vi "labview_master_02.vi"() -> ()   [LabVIEW 2018]
panel:
  out "Error Out 2":errorcluster caption="에러 출력"
  in  "Error In 2":errorcluster caption="에러 입력"
  out "Error Out":errorcluster caption="에러 출력"
  in  "Error In":errorcluster caption="에러 입력"
  in  "클러스터":cluster{"불리언":bool, "문자열":string, "숫자형 컨트롤":dbl}
  out "dimension 6":dbl[][][](array[numeric])
  out "dimension 5":dbl[][](array[numeric])
  out "dimension 4":dbl[](array[numeric])
  in  "dimension 3":dbl[][][](array[numeric])
  in  "dimension 2":dbl[][](array[numeric])
  in  "dimension 1":dbl[](array[numeric])
  in  "열거형":enum16{"Channel A", "Channel B", "Channel C"}(ring)
  in  "문자열":string
  in  "불리언":bool
  in  "정수":i32
  in  "부동소수점형":dbl
  # "사용자 인터페이스 구현"
  # "숫자"
  # "불리언"
  # "문자열"
  # "열거형"
  # "배열"
  # "클러스터"
  # "기본 클러스터"
  # "전부 control"
  # "module 만들기"
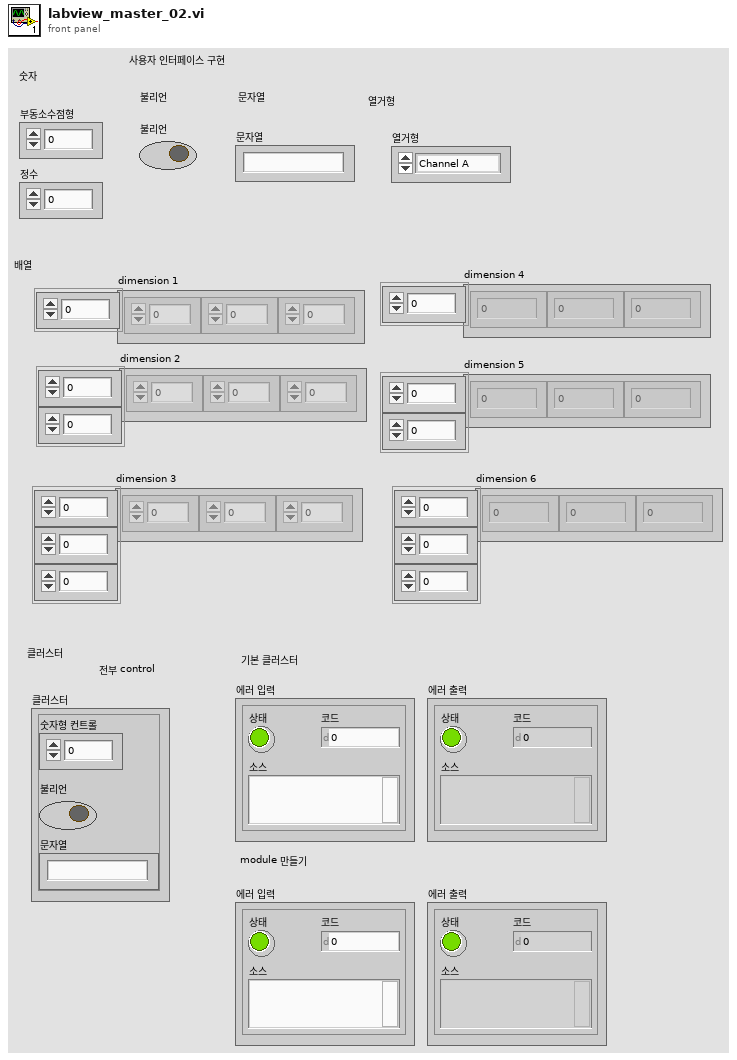
[diagram p1: front panel]
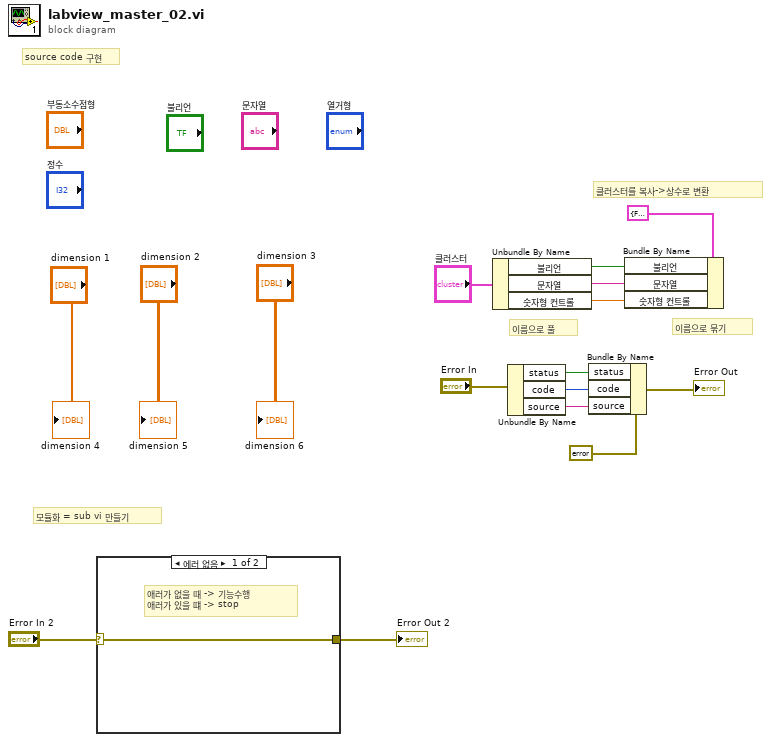
[diagram p0: block diagram]
diagram:
  # "모듈화 = sub vi 만들기"
  # "이름으로 풀"
  # "이름으로 묶기"
  # "클러스터를 복사->상수로 변환"
  # "source code 구현"
  n1 = case shown="에러 없음" "Error In 2" {
    selector: "Error In 2" -> [w17 _]
    tunnel: [w17 _] -> w1
    frame No Error {
      # "애러가 없을 때 -> 기능수행\n애러가 있을 떄 -> stop"
    }
    frame Error {
    }
  }
  "Error Out 2" <- w1
  n2 = Unbundle By Name("클러스터") -> ("불리언"=w11:bool, "문자열"=w10:string, "숫자형 컨트롤"=w9:dbl)
  n3 = Unbundle By Name("Error In") -> ("status"=w6:bool, "code"=w5:i32, "source"=w4:string)
  n4 = Bundle By Name(cluster=errorcluster {"status"=FALSE, "code"=0, "source"=""} ("Error In 2"), "status"=w6, "code"=w5, "source"=w4) -> (→"Error Out":errorcluster)
  n5 = Bundle By Name(cluster=cluster{"불리언":bool, "문자열":string, "숫자형 컨트롤":dbl} {"불리언"=FALSE, "문자열"="", "숫자형 컨트롤"=0.0} ("클러스터 2"), "불리언"=w11, "문자열"=w10, "숫자형 컨트롤"=w9) -> ()  [unwired: 1 out]
  "dimension 4" <- "dimension 1"
  "dimension 5" <- "dimension 2"
  "dimension 6" <- "dimension 3"
